vi "new algo test.vi"() -> ()   [LabVIEW 2026]
uses:
  <vilib>/FPGAPlugInAG/cRIO-9047/niLvFpga_Open_cRIO-9047.vi
  <vilib>/FPGAPlugInAG/cRIO-9047/niLvFpga_Run_cRIO-9047.vi
  <vilib>/Utility/error.llb/Error Cluster From Error Code.vi
  <vilib>/rvi/errors/niLvFpgaAdjustHostInterfaceError.vi
  <vilib>/rvi/interface/nirviOpenFPGA/nirviOpenFPGA.xnode
  FPGA Bitfiles/speedofvight_FPGATarget_DetectionLogicto_z92qlUcGACA.lvbitx
  <vilib>/rvi/interface/nirviMethod/nirviMethod.xnode
  <vilib>/rvi/interface/nirviReadWriteControl/nirviReadWriteControl.xnode
  NiFpgaLv.dll
panel:
  in  "stop":bool
  out "Pressed":bool[][](array[boolean])
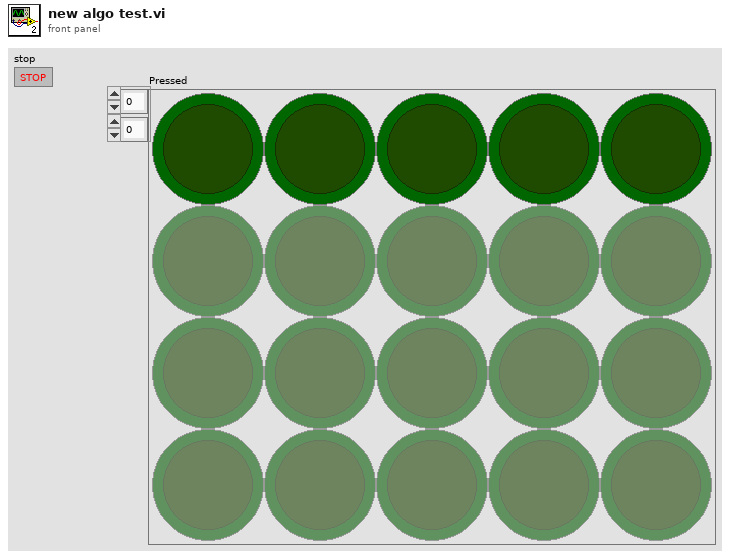
[diagram p1: front panel]
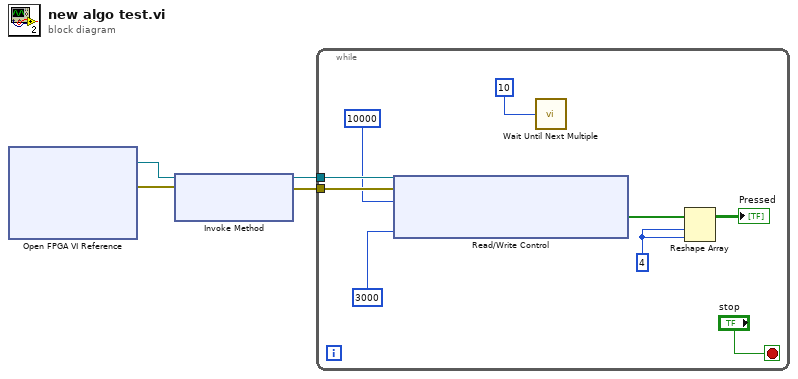
[diagram p0: block diagram]
diagram:
  n1 = xnode "Open FPGA VI Reference"() -> ("FPGA VI Reference Out"=w3:refnum<k20>, "error out"=w4:errorcluster)  [unwired: 2 in]
  n2 = xnode "Invoke Method"("FPGA VI Reference In"=w3, "error in"=w4) -> ("FPGA VI Reference Out"=w1:refnum<k20>, "error out"=w2:errorcluster)  [unwired: 1 in]
  n3 = while {
    tunnel: w2 -> [w13]
    tunnel: w1 -> [w12]
    stop <- "stop" stop-if-true
    w5 = 4 ("dimension size")
    n4 = xnode "Read/Write Control"("FPGA VI Reference In"=w12, "error in"=w13, "Speed Threshold, ticks"=u64 10000, "Debounce Threshold, ticks"=u64 3000) -> ("Pressed"=w11:bool[])  [unwired: 2 out]
    n5 = call "Wait Until Next Multiple"("Count(mSec)"=u32 10 ("Count(Ticks)")) -> ()  [unwired: 1 out]
    n6 = Reshape Array(w11, w5, w5) -> (→"Pressed":bool[][])
  }
